vi "S8.vi"(1 "Input array":bool[](array[boolean])) -> (0 "Array":bool[](array[boolean]))   [LabVIEW 2013]
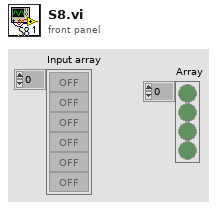
[diagram p1: front panel]
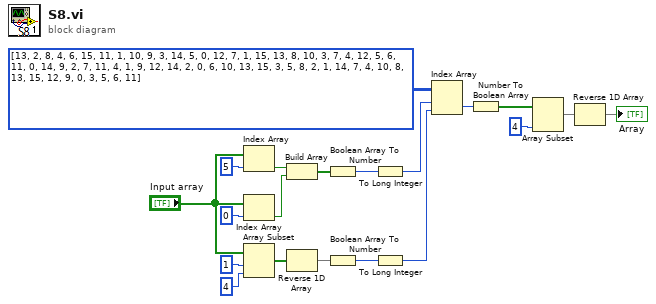
[diagram p0: block diagram]
diagram:
  n1 = Index Array(array="Input array", index=5) -> (element=w4:bool)
  n2 = Index Array(array="Input array", index=0) -> (element=w3:bool)
  n3 = Array Subset(array="Input array", index=1, length=4) -> (w10:bool[])
  n4 = Build Array(w4, w3) -> (w1:bool[])
  n5 = Reverse 1D Array(array=w10) -> (reversed array=w9:bool[])
  n6 = Boolean Array To Number(Boolean array=w1) -> (number=w14:u32)
  n7 = Boolean Array To Number(Boolean array=w9) -> (number=w13:u32)
  n8 = To Long Integer(number=w14) -> (32bit integer=w8:i32)
  n9 = To Long Integer(number=w13) -> (32bit integer=w7:i32)
  n10 = Index Array(array=u8[][] [[13, 2, 8, 4, 6, 15, 11, 1, 10, 9, 3, 14, 5, 0, 12, 7], [1, 15, 13, 8, 10, 3, 7, 4, 12, 5, 6, 11, 0, 14, 9, 2], [7, 11, 4, 1, 9, 12, 14, 2, 0, 6, 10, 13, 15, 3, 5, 8], [2, 1, 14, 7, 4, 10, 8, 13, 15, 12, 9, 0, 3, 5, 6, 11]], index (row)=w8, index (col)=w7) -> (element=w19:u8)
  n11 = Number To Boolean Array(number=w19) -> (Boolean array=w18:bool[])
  n12 = Array Subset(array=w18, length=4) -> (w6:bool[])  [unwired: 1 in]
  n13 = Reverse 1D Array(array=w6) -> (reversed array=→"Array":bool[])
